vi "stdin.vi"() -> (0 "stdin":path)   [LabVIEW 2014]
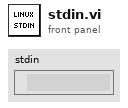
[diagram p1: front panel]
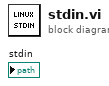
[diagram p0: block diagram]
diagram:
